vi "其他禁用读取 9.vi"(4 "error in (no error)":errorcluster caption="错误输入（无错误）", 6 "Container State":T2 caption="容器状态", 7 "Display State In":T1={"模块启用"={"河水净化禁用"=enum."Enabled", "采配水禁用"=enum."Enabled", "氨氮禁用"=enum."Enabled", "总磷总氮禁用"=enum."Enabled", "总氮禁用"=enum."Enabled", "多参数禁用"=enum."Enabled", "CODMn禁用"=enum."Enabled", "CODcr禁用"=enum."Enabled", "流量计禁用"=enum."Enabled", "质控单元禁用"=enum."Enabled", "超标留样禁用"=enum."Enabled", "其他禁用"=enum."Enabled"}, "模块名称"={"氨氮模块名称"="氨氮", "总磷总氮模块名称"="总磷总氮"}} caption="显示状态输入") -> (0 "error out":errorcluster caption="错误输出", 2 "Value":T3(ring) caption="值", 3 "Display State Out":T1={"模块启用"={"河水净化禁用"=enum."Enabled", "采配水禁用"=enum."Enabled", "氨氮禁用"=enum."Enabled", "总磷总氮禁用"=enum."Enabled", "总氮禁用"=enum."Enabled", "多参数禁用"=enum."Enabled", "CODMn禁用"=enum."Enabled", "CODcr禁用"=enum."Enabled", "流量计禁用"=enum."Enabled", "质控单元禁用"=enum."Enabled", "超标留样禁用"=enum."Enabled", "其他禁用"=enum."Enabled"}, "模块名称"={"氨氮模块名称"="氨氮", "总磷总氮模块名称"="总磷总氮"}} caption="显示状态输出")   [LabVIEW 2016, in "运维调试菜单.xctl"]
uses:
  <vilib>/_xctls/Container State.ctl
  <vilib>/_xctls/XControlSupport.lvlib
panel:
  # "将以下值显示控件替换为所需类型的显示控件。\n不要从连线板中删除该显示控件或其它显示控件。\n不要更改连线板模式。\n值显示控件应始终位于连线板输出端自顶部起第二个接线端。"
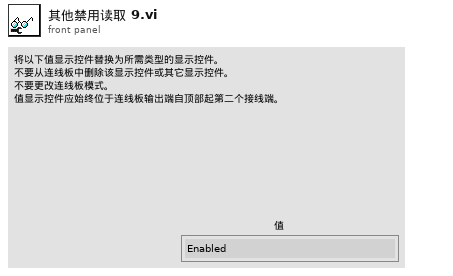
[diagram p1: front panel]
types:
  T1 = typedef "运维调试菜单.xctl/状态 1.ctl" = cluster{"模块启用":cluster{"河水净化禁用":enum16{"Enabled", "Disabled", "Disabled and Grayed Out"}, "采配水禁用":enum16{"Enabled", "Disabled", "Disabled and Grayed Out"}, "氨氮禁用":enum16{"Enabled", "Disabled", "Disabled and Grayed Out"}, "总磷总氮禁用":enum16{"Enabled", "Disabled", "Disabled and Grayed Out"}, "总氮禁用":enum16{"Enabled", "Disabled", "Disabled and Grayed Out"}, "多参数禁用":enum16{"Enabled", "Disabled", "Disabled and Grayed Out"}, "CODMn禁用":enum16{"Enabled", "Disabled", "Disabled and Grayed Out"}, "CODcr禁用":enum16{"Enabled", "Disabled", "Disabled and Grayed Out"}, "流量计禁用":enum16{"Enabled", "Disabled", "Disabled and Grayed Out"}, "质控单元禁用":enum16{"Enabled", "Disabled", "Disabled and Grayed Out"}, "超标留样禁用":enum16{"Enabled", "Disabled", "Disabled and Grayed Out"}, "其他禁用":enum16{"Enabled", "Disabled", "Disabled and Grayed Out"}}, "模块名称":cluster{"氨氮模块名称":string, "总磷总氮模块名称":string}}
  T2 = typedef "XControlSupport.lvlib/Container State.ctl" = cluster{"Indicator?":bool, "Run Mode?":bool, " Refnum":refnum<vi>}
  T3 = enum16{"Enabled", "Disabled", "Disabled and Grayed Out"}
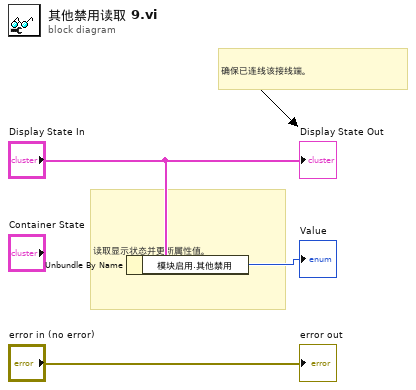
[diagram p0: block diagram]
diagram:
  # "确保已连线该接线端。"
  # "读取显示状态并更新属性值。"
  n1 = Unbundle By Name("Display State In") -> ("模块启用.其他禁用"=→"Value":T3)
  "error out" <- "error in (no error)"
  "Display State Out" <- "Display State In"
